vi "set channel.vi"(8 "error in":errorcluster, 10 "channel":refnum<class "TBM channel.lvclass">, 11 "Scaling configuration in":refnum<class "Scaling configuration.lvclass">) -> (0 "error out":errorcluster, 3 "Scaling configuration out":refnum<class "Scaling configuration.lvclass">)   [LabVIEW 2013, in "Scaling configuration.lvclass"]
doc: "This function is responsible for replacing a channel, by name in the configuration class."
uses:
  Scaling configuration.lvclass
  <vilib>/NI/Tag Bus/tag/tag descriptor.lvclass
  <vilib>/NI/Tag Bus Module Framework/channel/TBM channel.lvclass
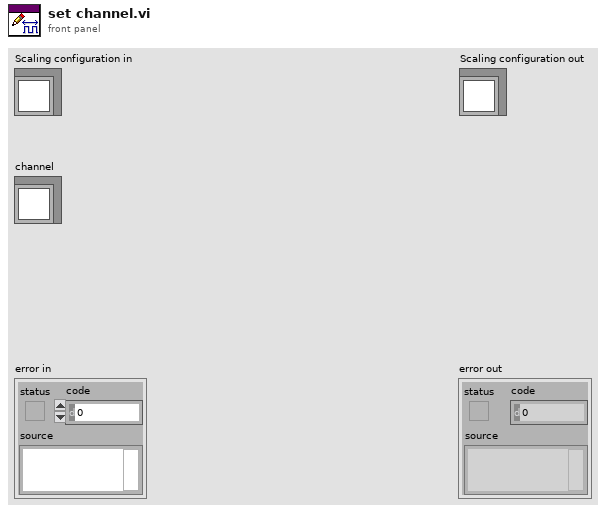
[diagram p1: front panel]
types:
  T1 = typedef "Scaling configuration.lvclass/scale data types.ctl" = enum16{"Double", "Single", "I64", "I32", "I16", "I8", "U64", "U32", "U16", "U8"}
  T2 = cluster{"input channel":refnum<class "TBM channel.lvclass">, "output channel":refnum<class "TBM channel.lvclass">, "input data type":T1, "output data type":T1}[][]
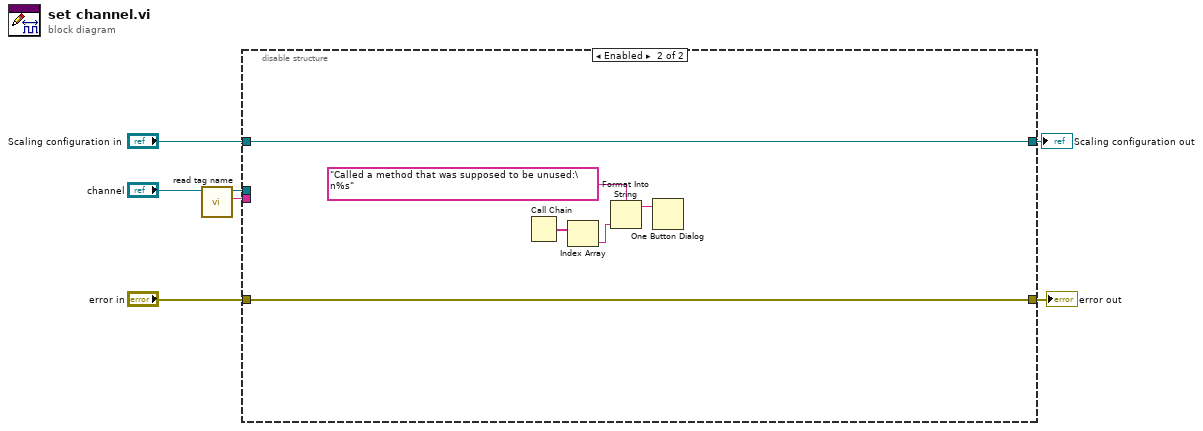
[diagram p0: block diagram]
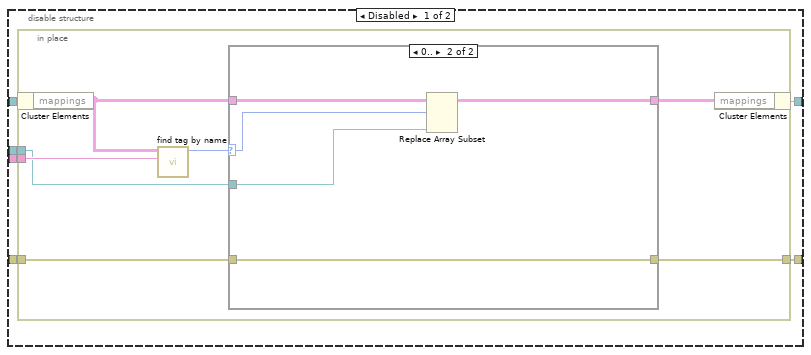
[diagram p2: hidden frame]
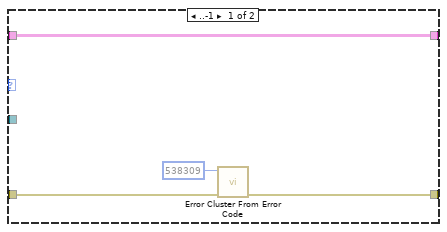
[diagram p3: hidden frame]
diagram:
  n1 = call <vilib>:"read tag name.vi"("system tag in"="channel") -> ("name"=w6:string, "system tag out"=w7:refnum<class "TBM channel.lvclass">)  [unwired: 8 in, 1 out]
  n2 = disable-structure shown="Enabled" {
    disable-tunnel: w7 -> [w13 _]
    disable-tunnel: w6 -> [w12 _]
    disable-tunnel: [w11 w35] -> w5
    disable-tunnel: [w10 w34] -> w4
    disable-tunnel: "Scaling configuration in" -> [w9 w35]
    disable-tunnel: "error in" -> [w8 w34]
    frame Disabled {
      n3 = in-place {
        in-place-border: [w19] -> w10
        in-place-border: w8 -> [w17]
        in-place-border: w13 -> [w15]
        in-place-border: w12 -> [w16]
        n4 = in-place-cluster #1(w9) -> ("mappings"=w20:T2)
        n5 = call <vilib>:"find tag by name.vi"("name"=w16, "tags in"=w20) -> ("index"=w14:i32)  [unwired: 9 in]
        n6 = case shown="0.." w14 {
          selector: w14 -> [_ w25]
          tunnel: w20 -> [w22 w28]
          tunnel: [w23 w29] -> w19
          tunnel: [w22 w27] -> w18
          tunnel: w17 -> [w21 w29]
          tunnel: w15 -> [_ w26]
          frame ..-1 {
            n7 = call <vilib>:"Error Cluster From Error Code.vi"("error in (no error)"=w21, "error code (0)"=538309) -> ("error out"=w23:errorcluster)  [unwired: 7 in]
          }
          frame 0.. {
            n8 = Replace Array Subset(array=w28, new element=w26, index (row)=w25) -> (w27:T2)  [unwired: 1 in]
          }
        }
        n9 = in-place-cluster #1("mappings"=w18) -> (w11:refnum<class "Scaling configuration.lvclass">)
      }
    }
    frame Enabled {
      n10 = Call Chain() -> (call chain=w33:string[])
      n11 = Index Array(array=w33) -> (element=w31:string)  [unwired: 1 in]
      n12 = Format Into String(format string="Called a method that was supposed to be unused:\n%s", w31) -> (resulting string=w30:string)  [unwired: 2 in, 1 out]
      n13 = One Button Dialog(message=w30) -> ()  [unwired: 1 in, 1 out]
    }
  }
  "error out" <- w4
  "Scaling configuration out" <- w5
